vi "Log Event.vi"(7 "Event Level":T1, 8 "error in (no error)":errorcluster, 10 "Event":string, 11 "Network Session Handler in":refnum<class "Network Session Handler.lvclass">) -> (0 "error out":errorcluster, 3 "Network Session Handler out":refnum<class "Network Session Handler.lvclass">)   [LabVIEW 2017, in "Network Interface.lvlib" / "Network Session Handler.lvclass"]
uses:
  <vilib>/gpm_packages/@cs/Network-sink/Source/Network Interface/Network Session Handler/Network Session Handler.lvclass
  <vilib>/gpm_packages/@cs/event-logger/Source/Composed Log/Types/Log Level.ctl
  <vilib>/gpm_packages/@cs/Network-sink/Source/Network Interface/Network Session Handler/Network Session Handler.lvclass/Network Session Handler.ctl
  <vilib>/gpm_packages/@cs/event-logger/Source/Composed Log/LoggerReference/LoggerReference.lvclass/LoggerReference.ctl
  <vilib>/gpm_packages/@cs/event-logger/Source/Composed Log/LoggerReference/Log.vi
  <vilib>/gpm_packages/@cs/event-logger/Source/Composed Log/LoggerReference/Get Valid Event Time.vi
  <vilib>/gpm_packages/@cs/event-logger/Source/Composed Log/LoggerReference/Remove Stale Logs.vi
  <vilib>/gpm_packages/@cs/event-logger/Source/Composed Log/LoggerReference/LoggerReference.lvclass
  <vilib>/gpm_packages/@cs/event-logger/Source/Composed Log/Composed Log.lvlib
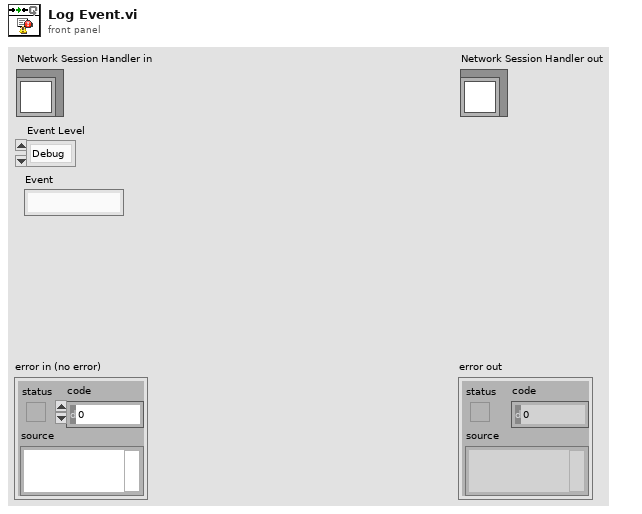
[diagram p1: front panel]
types:
  T1 = typedef "Composed Log.lvlib/Log Level.ctl" = enum16{"Debug", "Info", "Warning", "Error", "Critical"}
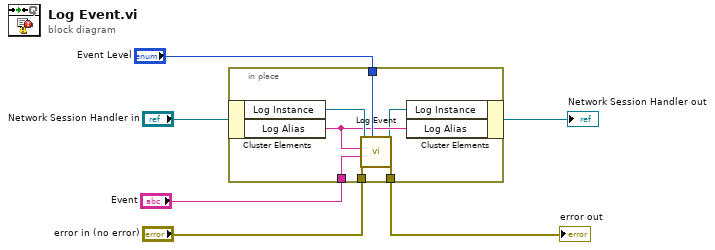
[diagram p0: block diagram]
diagram:
  n1 = in-place {
    in-place-border: "Event Level" -> [w13]
    in-place-border: "Event" -> [w12]
    in-place-border: "error in (no error)" -> [w8]
    in-place-border: [w7] -> w1
    n2 = in-place-cluster #1("Network Session Handler in") -> ("Log Instance"=w11:refnum<class "LoggerReference.lvclass">, "Log Alias"=w10:string)
    n3 = call <vilib>:"Log Event.vi"("Event Level"=w13, "error in (no error)"=w8, "Data To Log"=w12, "SourceID"=w10, "Log Instance"=w11) -> ("error out"=w7:errorcluster, "Log Instance Out"=w9:refnum<class "LoggerReference.lvclass">)  [unwired: 5 in]
    n4 = in-place-cluster #1("Log Instance"=w9, "Log Alias"=w10) -> (→"Network Session Handler out":refnum<class "Network Session Handler.lvclass">)
  }
  "error out" <- w1
